vi "Interval Array.vi"(9 "Interval":sgl, 10 "Min":sgl, 11 "Max":sgl) -> (3 "Level Array":sgl[](array[numeric]))   [LabVIEW 2020, in "3D Contour.lvclass"]
uses:
  <vilib>/Math Plots/3D Math Plots/3D Contour/3D Contour/3D Contour.lvclass
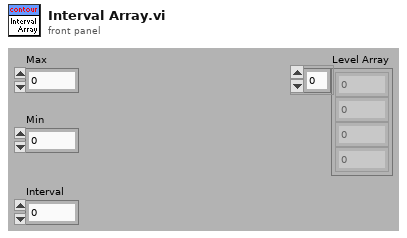
[diagram p1: front panel]
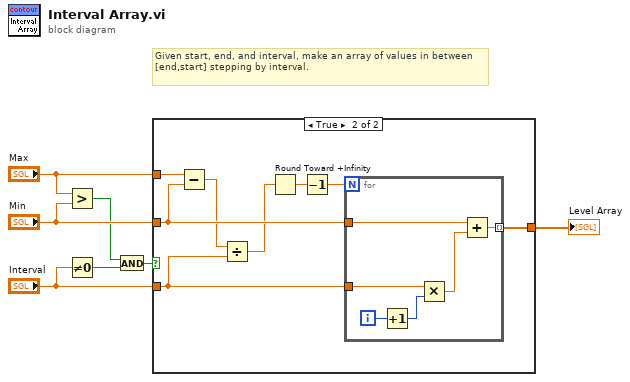
[diagram p0: block diagram]
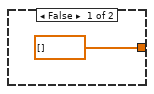
[diagram p2: hidden frame]
diagram:
  # "Given start, end, and interval, make an array of values in between [end,start] stepping by interval."
  n1 = Greater?(x="Max", y="Min") -> (0:w2:bool)
  n2 = Not Equal To 0?(x="Interval") -> (x != 0?=w3:bool)
  n3 = And(x=w2, y=w3) -> (x .and. y?=w1:bool)
  n4 = case shown="True" w1 {
    tunnel: "Max" -> [_ w16]
    tunnel: "Interval" -> [_ w13]
    tunnel: "Min" -> [_ w15]
    tunnel: [sgl[] [] w14] -> w7
    frame False {
    }
    frame True {
      n5 = Subtract(x=w16, y=w15) -> (x-y=w12:sgl)
      n6 = Divide(x=w12, y=w13) -> (x/y=w11:sgl)
      n7 = Round Toward +Infinity(x=w11) -> (ceil(x): smallest int >= x=w10:sgl)
      n8 = Decrement(x=w10) -> (x-1=w9:sgl)
      n9 = for {
        N: w9 -> [_]
        tunnel: w13 -> [w22]
        tunnel: w15 -> [w20]
        tunnel: [w19] -> w14 mode=indexing
        i -> [w18]
        n10 = Increment(x=w18) -> (x+1=w17:i32)
        n11 = Multiply(x=w22, y=w17) -> (x*y=w21:sgl)
        n12 = Add(x=w20, y=w21) -> (x+y=w19:sgl)
      }
    }
  }
  "Level Array" <- w7
